vi "High Throughput Streaming - From Disk (Host).vi"() -> ()   [LabVIEW 2016]
doc: "Example Description:\nGenerates data at the specified rate from disk to a RIO device using TDMS asynchronous reads instead of the built-in LabVIEW file I/O.\n\nAsynchronous reads provide for the best possible performance, since the HDD controller can spend more time transferring data than is possible with synchronous blocking reads. Furthermore, since TDMS effectively queues up the data from multiple reads for us, queues on the LabVEIW diagram are no longer necessary, simplifying the application by removing the queue and the separate read and write loops.\n\nVI Configuration:\nThis example uses the PXI-7966R as the FPGA target by default. To use this VI with another FPGA target, use the following steps to configure the host VI to use a VI configured for your FPGA target:\n\n1. On the block diagram, right-click the Open FPGA VI Reference (PXI-7966R) VI and select Configure Open FPGA VI Reference.\n2. Browse for a new target by clicking the Browse Project button in the Open VI section.\n3. Select the VI under the target that matches your device. Click OK to select this VI.\n4. Click OK to exit the dialog box and to apply the new selection to the FPGA VI.\n\nRunning the VI:\n1. Select a RIO Resource that corresponds to the FPGA device configured above.\n2. Select a source TDMS file that you will be streaming data from.\n3. Configure the Requested host Buffer Depth, Write Size, Max TDMS Asynchronous Reads, and Requested (M) controls on the Host VI Front Panel.\n4. Click the run arrow to run the VI.\n5. Observe the Status of the Host Buffer as well as the Output DMA FIFO.\n6. Observe the achieved Streaming Throughput.\n7. Click Stop on the Front Panel to stop the example\n\n\nExecution Steps:\nRefer to the block diagram of the Host VI for each example to view the execution steps for that specific example."
uses:
  <vilib>/userdefined/High Color/nirio_resource_hc.ctl
  <vilib>/FPGAPlugInAG/PXIe-7966R/niLvFpga_Open_PXIe-7966R.vi
  <vilib>/rvi/interface/common/dynamic/niFpgaDynamicAddResources.vi
  <vilib>/Utility/error.llb/Error Cluster From Error Code.vi
  <vilib>/rvi/errors/niLvFpgaAdjustHostInterfaceError.vi
  <vilib>/FPGAPlugInAG/Dynamic/niLvFpga_Run_Dynamic.vi
  <vilib>/rvi/interface/common/niFpgaWaitOnOcc.vi
  <vilib>/FPGAPlugInAG/Dynamic/niLvFpga_Close_Dynamic.vi
  <vilib>/rvi/interface/nirviOpenFPGA/nirviOpenFPGA.xnode
  FPGA Bitfiles/HighThroug_PXIe-7966R.lvbitx
  <vilib>/rvi/interface/nirviReadWriteControl/nirviReadWriteControl.xnode
  <vilib>/rvi/interface/nirviMethod/nirviMethod.xnode
  <vilib>/rvi/interface/nirviCloseFPGA/nirviCloseFPGA.xnode
  <vilib>/rvi/interface/Simulation/niFpgaSimulationCallBeginRW.vi
  <vilib>/FPGAPlugInAG/Dynamic/niLvFpga_AcquireWriteRegionFifo_Dynamic.vi
  <vilib>/rvi/errors/niLvFpgaMergeErrorWithErrorCode.vi
  NiFpgaLv.dll
  <vilib>/FPGAPlugInAG/Dynamic/niLvFpga_ConfigureFifo_Dynamic.vi
panel:
  out "Pending TDMS Reads":u32 caption="Pending"
  out "Max Pending TDMS Reads":u32 caption="Max Pending"
  out "output.Max Throughput":u16 caption="Maximum (M)"
  in  "Requested Throughput":u16=1000 caption="Requested (M)" step=5
  out "output.Ever Timed Out?":bool caption="Underflow"
  out "error out":errorcluster
  in  "Stop":bool
  in  "Max TMDS Asynchronous Reads":u32=8
  out "Generation Size (samples)":u64
  out "Host Buffer Depth (samples)":u32
  out "Host Buffer Status":cluster{u32, u32, u32}(slide) scale=0.0..67108864.0 scale format="%#.1p"
  in  "Requested Host Buffer Depth (samples)":u32=67108864 step=1048576
  in  "Write Size (samples)":u32=4194304 step=1048576
  in  "file path":path=path "Select a source TDMS file"
  out "Stop...":bool
  out "output.Throughput (B/s)":dbl caption="Actual" format="%#.1p"
  in  "output.Reset":bool
  out "output.FPGA FIFO Status":cluster{u32, u32}(slide) caption="FIFO Status" scale=0.0..65559.0 scale format="%#.1p"
  out "Samples Generated":u64(slide) caption="Generation Progress" scale=0.0..1000000000.0 scale format="%#.1p"
  in  "resource name":T1="Select RIO resource"
  # "Configuration"
  # "Host"
  # "TDMS Reads"
  # "Output FPGA"
  # "Throughput (B/s)"
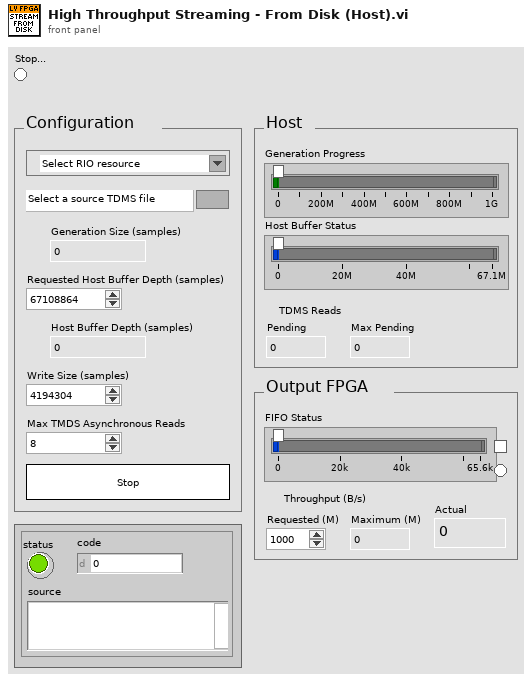
[diagram p1: front panel]
types:
  T1 = typedef "nirio_resource_hc.ctl" = tag
  T2 = enum16{"open", "open or create", "create or replace", "create", "open (read-only)"}
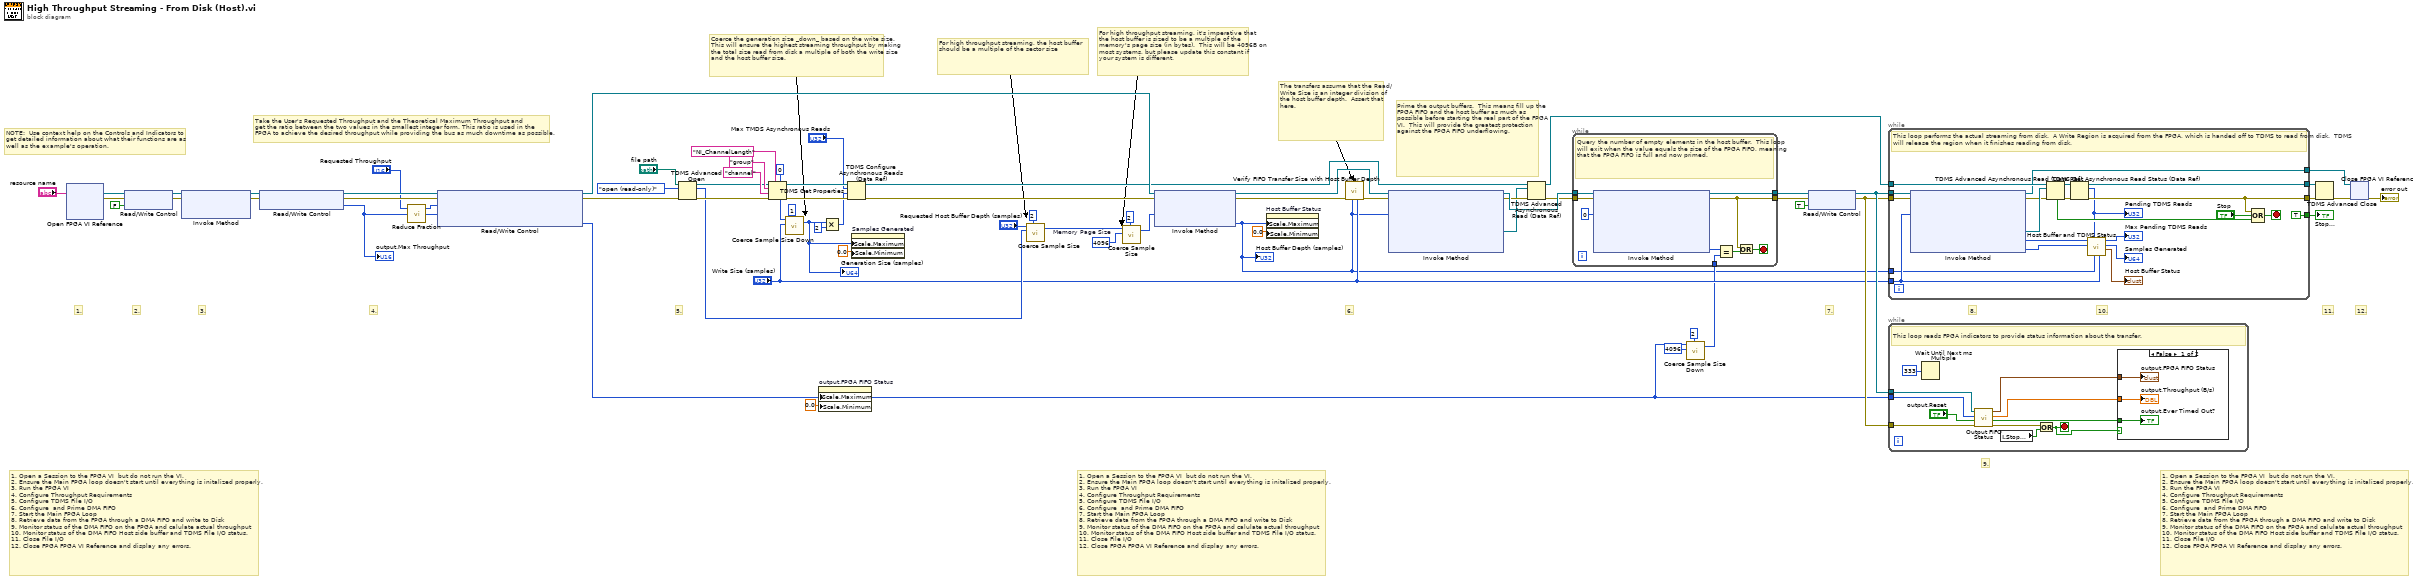
[diagram p0: block diagram]
diagram:
  w35 = u64 4096  # Memory Page Size
  # "1. Open a Session to the FPGA VI  but do not run the VI.\n2. Ensure the Main FPGA loop doesn't start until everything is initalized properly. \n3. Run the FPGA VI\n4. Configure Throughput Requirements\n5. Configure TDMS File I/O\n6. Configure  and Prime DMA FIFO\n7. Start the Main FPGA Loop\n8. Retrieve data from the FPGA through a DMA FIFO and write to Disk\n9. Monitor status of the DMA FIFO on the FPGA and calulate actual throughput\n10. Monitor status of the DMA FIFO Host side buffer and TDMS File I/O status.\n11. Close File I/O\n12. Close FPGA FPGA VI Reference and display any errors."
  # "1. Open a Session to the FPGA VI  but do not run the VI.\n2. Ensure the Main FPGA loop doesn't start until everything is initalized properly. \n3. Run the FPGA VI\n4. Configure Throughput Requirements\n5. Configure TDMS File I/O\n6. Configure  and Prime DMA FIFO\n7. Start the Main FPGA Loop\n8. Retrieve data from the FPGA through a DMA FIFO and write to Disk\n9. Monitor status of the DMA FIFO on the FPGA and calulate actual throughput\n10. Monitor status of the DMA FIFO Host side buffer and TDMS File I/O status.\n11. Close File I/O\n12. Close FPGA FPGA VI Reference and display any errors."
  # "12."
  # "11."
  # "Take the User's Requested Throughput and the Theoretical Maximum Throughput and\nget the ratio between the two values in the smallest integer form. This ratio is used in the \nFPGA to achieve the desired throughput while providing the bus as much downtime as possible."
  # "1. Open a Session to the FPGA VI  but do not run the VI.\n2. Ensure the Main FPGA loop doesn't start until everything is initalized properly. \n3. Run the FPGA VI\n4. Configure Throughput Requirements\n5. Configure TDMS File I/O\n6. Configure  and Prime DMA FIFO\n7. Start the Main FPGA Loop\n8. Retrieve data from the FPGA through a DMA FIFO and write to Disk\n9. Monitor status of the DMA FIFO on the FPGA and calulate actual throughput\n10. Monitor status of the DMA FIFO Host side buffer and TDMS File I/O status.\n11. Close File I/O\n12. Close FPGA FPGA VI Reference and display any errors."
  # "9."
  # "7."
  # "10."
  # "8."
  # "6."
  # "5."
  # "4."
  # "3."
  # "2."
  # "1."
  # "NOTE:  Use context help on the Controls and Indicators to \nget detailed information about what their functions are as\nwell as the example's operation."
  # "For high throughput streaming, the host buffer should be a multiple of the sector size"
  # "Coerce the generation size _down_ based on the write size.  This will ensure the highest streaming throughput by making the total size read from disk a multiple of both the write size and the host buffer size."
  # "For high throughput streaming, it's imperative that the host buffer is sized to be a multiple of the memory's page size (in bytes).  This will be 4096B on most systems, but please update this constant if your system is different."
  # "The transfers assume that the Read/Write Size is an integer division of the host buffer depth.  Assert that here."
  # "Prime the output buffers.  This means fill up the FPGA FIFO and the host buffer as much as possible before starting the real part of the FPGA VI.  This will provide the greatest protection against the FPGA FIFO underflowing."
  n1 = xnode "Open FPGA VI Reference"("resource name"="resource name") -> ("FPGA VI Reference Out"=w62:refnum<k20>, "error out"=w61:errorcluster)  [unwired: 1 in]
  n2 = xnode "Read/Write Control"("FPGA VI Reference In"=w62, "error in"=w61, "output.Start"=FALSE) -> ("FPGA VI Reference Out"=w60:refnum<k20>, "error out"=w59:errorcluster)
  n3 = xnode "Invoke Method"("FPGA VI Reference In"=w60, "error in"=w59) -> ("FPGA VI Reference Out"=w10:refnum<k20>, "error out"=w9:errorcluster)  [unwired: 1 in]
  n4 = xnode "Read/Write Control"("FPGA VI Reference In"=w10, "error in"=w9) -> ("FPGA VI Reference Out"=w7:refnum<k20>, "error out"=w8:errorcluster, "output.Max Throughput"=w5:u16)
  "output.Max Throughput" <- w5
  n5 = call "Reduce Fraction.vi"("denominator"=w5, "numerator"="Requested Throughput") -> ("reduced denominator"=w6:u16, "reduced numerator"=w3:u16)  [unwired: 2 in]
  n6 = xnode "Read/Write Control"("FPGA VI Reference In"=w7, "error in"=w8, "output.Requested Throughput"=w3, "output.Requested Throughput Denominator"=w6) -> ("FPGA VI Reference Out"=w29:refnum<k20>, "error out"=w49:errorcluster, "output.FIFO Size"=w13:u32)
  n7 = TDMS Advanced Open(8:w49, 10:T2."open (read-only)" ("operation (0:open)"), 11:"file path") -> (0:w46:errorcluster, 2:w31:u32, 3:w44:refnum<k34>)  [unwired: 2 in]
  n8 = TDMS Get Properties(5:u64 0, 7:"NI_ChannelLength" ("property name"), 8:w46, 9:"channel" ("channel name"), 10:"group" ("group name"), 11:w44) -> (0:w45:errorcluster, 3:w43:refnum<k34>, 4:w40:u64)  [unwired: 3 out]
  n9 = call "Coerce Sample Size Down.vi"("Bytes Per Sample (B)"=u64 1, "Coerce To (B)"="Write Size (samples)", "Size (samples)"=w40) -> ("Coerced Size (samples)"=w1:u64)  [unwired: 4 in]
  "Generation Size (samples)" <- w1
  n10 = property on="output.FPGA FIFO Status" class="Slide (strict)"("Scale.Maximum"=w13, "Scale.Minimum"=0.0 ("Scale.Range:Minimum")) -> ()  [unwired: 2 in, 2 out]
  n11 = Multiply(x=w1, y=u64 2 ("Bytes per Sample")) -> (x*y=w39:u64)
  n12 = TDMS Configure Asynchronous Reads (Data Ref)(8:w45, 9:w39, 10:"Max TMDS Asynchronous Reads", 11:w43) -> (0:w30:errorcluster, 3:w21:refnum<k34>)  [unwired: 1 in]
  n13 = property on="Samples Generated" class="Slide (strict)"("Scale.Maximum"=w1, "Scale.Minimum"=0.0 ("Scale.Range:Minimum")) -> ()  [unwired: 2 in, 2 out]
  n14 = call "Coerce Sample Size.vi"("Bytes Per Sample (B)"=u64 2, "Coerce To (B)"=w31, "Size (samples)"="Requested Host Buffer Depth (samples)") -> ("Coerced Size (samples)"=w36:u64)  [unwired: 4 in]
  n15 = call "Coerce Sample Size.vi"("Bytes Per Sample (B)"=u64 2, "Coerce To (B)"=w35, "Size (samples)"=w36) -> ("Coerced Size (samples)"=w28:u64)  [unwired: 4 in]
  n16 = xnode "Invoke Method"("FPGA VI Reference In"=w29, "error in"=w30, "Requested Depth"=w28) -> ("FPGA VI Reference Out"=w20:refnum<k20>, "error out"=w23:errorcluster, "Actual Depth"=w2:u32)
  "Host Buffer Depth (samples)" <- w2
  n17 = property on="Host Buffer Status" class="Slide (strict)"("Scale.Maximum"=w2, "Scale.Minimum"=0.0 ("Scale.Range:Minimum")) -> ()  [unwired: 2 in, 2 out]
  n18 = call "Verify FIFO Transfer Size with Host Buffer Depth.vi"("Read/Write Size (samples)"="Write Size (samples)", "Host Buffer Depth (samples)"=w2, "error in"=w23) -> ("error out"=w22:errorcluster)  [unwired: 8 in]
  n19 = xnode "Invoke Method"("FPGA VI Reference In"=w20, "error in"=w22, "Number of Elements"=w2) -> ("FPGA VI Reference Out"=w69:refnum<k20>, "error out"=w26:errorcluster, "Write Region Reference"=w25:refnum<data-value>)  [unwired: 1 in, 2 out]
  n20 = TDMS Advanced Asynchronous Read (Data Ref)(8:w26, 10:w25, 11:w21) -> (0:w24:errorcluster, 3:w16:refnum<k34>)  [unwired: 1 in, 1 out]
  n21 = call "Coerce Sample Size Down.vi"("Bytes Per Sample (B)"=u64 2, "Coerce To (B)"=u64 4096, "Size (samples)"=w13) -> ("Coerced Size (samples)"=w14:u64)  [unwired: 4 in]
  n22 = while {
    tunnel: w24 -> [w78]
    tunnel: [w75] -> w18
    tunnel: w69 -> [w77]
    tunnel: w14 -> [w73]
    tunnel: [w70] -> w17
    stop <- w76 stop-if-true
    # "Query the number of empty elements in the host buffer.  This loop will exit when the value equals the size of the FPGA FIFO, meaning that the FPGA FIFO is full and now primed."
    n23 = xnode "Invoke Method"("FPGA VI Reference In"=w77, "error in"=w78, "Number of Elements"=u32 0) -> ("FPGA VI Reference Out"=w70:refnum<k20>, "error out"=w75:errorcluster, "Empty Elements Remaining"=w71:u32)  [unwired: 1 in, 2 out]
    n24 = Equal?(x=w71, y=w73) -> (x = y?=w74:bool)
    n25 = Or(x=w75, y=w74) -> (x .or. y?=w76:bool)
  }
  n26 = xnode "Read/Write Control"("FPGA VI Reference In"=w17, "error in"=w18, "output.Start"=TRUE ("Start")) -> ("FPGA VI Reference Out"=w55:refnum<k20>, "error out"=w54:errorcluster)
  n27 = while {
    tunnel: w55 -> [w100]
    tunnel: w16 -> [w99]
    tunnel: w54 -> [w98]
    tunnel: [w91] -> w67
    tunnel: "Write Size (samples)" -> [w80]
    tunnel: [TRUE] -> w63
    tunnel: [w89] -> w57
    tunnel: [w85] -> w15
    tunnel: w2 -> [w79]
    stop <- w97 stop-if-true
    # "This loop performs the actual streaming from disk.  A Write Region is acquired from the FPGA, which is handed off to TDMS to read from disk.  TDMS will release the region when it finishes reading from disk."
    n28 = xnode "Invoke Method"("FPGA VI Reference In"=w100, "error in"=w98, "Number of Elements"=w80) -> ("FPGA VI Reference Out"=w85:refnum<k20>, "error out"=w95:errorcluster, "Write Region Reference"=w96:refnum<data-value>, "Elements In Region"=w84:u32, "Empty Elements Remaining"=w83:u32)  [unwired: 1 in]
    n29 = TDMS Advanced Asynchronous Read (Data Ref)(8:w95, 10:w96, 11:w99) -> (0:w92:errorcluster, 3:w90:refnum<k34>, 4:w93:bool)  [unwired: 1 in]
    n30 = TDMS Get Asynchronous Read Status (Data Ref)(8:w92, 11:w90) -> (0:w91:errorcluster, 2:w82:u32, 3:w89:refnum<k34>)
    "Pending TDMS Reads" <- w82
    n31 = call "Host Buffer and TDMS Status.vi"("Read/Write Size (samples)"=w80, "Initial Samples Transferred (0)"=w79, "Number of Pending Reads/Writes"=w82, "Elements Remaining"=w83, "Elements In Region"=w84) -> ("Host Buffer Status"=→"Host Buffer Status":cluster{u32, u32, u32}, "Samples Transferred"=→"Samples Generated":u64, "Running Max of TDMS Reads/Writes"=→"Max Pending TDMS Reads":u32)  [unwired: 4 in]
    n32 = Compound Arithmetic op=OR(w91, "Stop", w93) -> (w97:bool)
  }
  "Stop..." <- w63
  n33 = while {
    tunnel: w55 -> [w102]
    tunnel: w54 -> [w110]
    tunnel: w13 -> [w108]
    stop <- w101 stop-if-true
    # "This loop reads FPGA indicators to provide status information about the transfer."
    n34 = Wait Until Next ms Multiple(millisecond multiple=u32 333) -> ()  [unwired: 1 out]
    n35 = call "Output FIFO Status.vi"("error in"=w110, "output.Reset"="output.Reset", "output.FIFO Size"=w108, "FPGA VI Reference"=w102) -> ("error out"=w107:errorcluster, "output.Ever Timed Out?"=w105:bool, "output.Throughput (B/s)"=w104:dbl, "output.FPGA FIFO Status"=w103:cluster{u32, u32})  [unwired: 4 in]
    n36 = local read "Stop..."() -> (w106:bool)
    n37 = Or(x=w107, y=w106) -> (x .or. y?=w101:bool)
    n38 = case shown="False" w101 {
      tunnel: w105 -> [w114 _]
      tunnel: w104 -> [w113 _]
      tunnel: w103 -> [w112 _]
      frame False {
        "output.Throughput (B/s)" <- w113
        "output.Ever Timed Out?" <- w114
        "output.FPGA FIFO Status" <- w112
      }
      frame True {
      }
    }
  }
  n39 = TDMS Advanced Close(8:w67, 11:w57) -> (0:w66:errorcluster)  [unwired: 2 in, 1 out]
  n40 = xnode "Close FPGA VI Reference"("FPGA VI Reference In"=w15, "error in"=w66) -> ("error out"=→"error out":errorcluster)
